vi "AnotherCaller.vi"() -> ()   [LabVIEW 2020]
uses:
  <vilib>/FTP/ftp0.llb/FTP Session.ctl
  <vilib>/FTP/NI_FTP.lvlib
panel:
  in  "object":T1
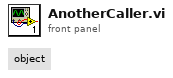
[diagram p1: front panel]
types:
  T1 = typedef "NI_FTP.lvlib/FTP Session.ctl" = refnum<k5>
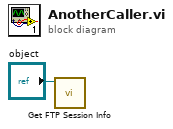
[diagram p0: block diagram]
diagram:
  n1 = call <vilib>:"Get FTP Session Info.vi"("object"="object") -> ()  [unwired: 6 in, 5 out]
